vi "Create (From GObject).vi"(8 "error in (no error)":errorcluster, 10 "GObject":refnum<vi>) -> (0 "error out":errorcluster, 1 "Structure Found in":refnum<vi>, 2 "Found JKI SMs?":bool, 3 "JKI SM out":refnum<class "JKI SM.lvclass">)   [LabVIEW 2020, in "JKI State Machine API.lvlib" / "JKI SM.lvclass"]
uses:
  JKI SM.lvclass
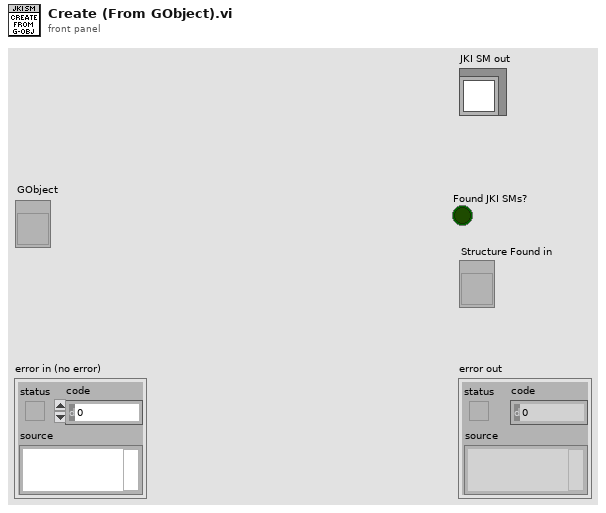
[diagram p1: front panel]
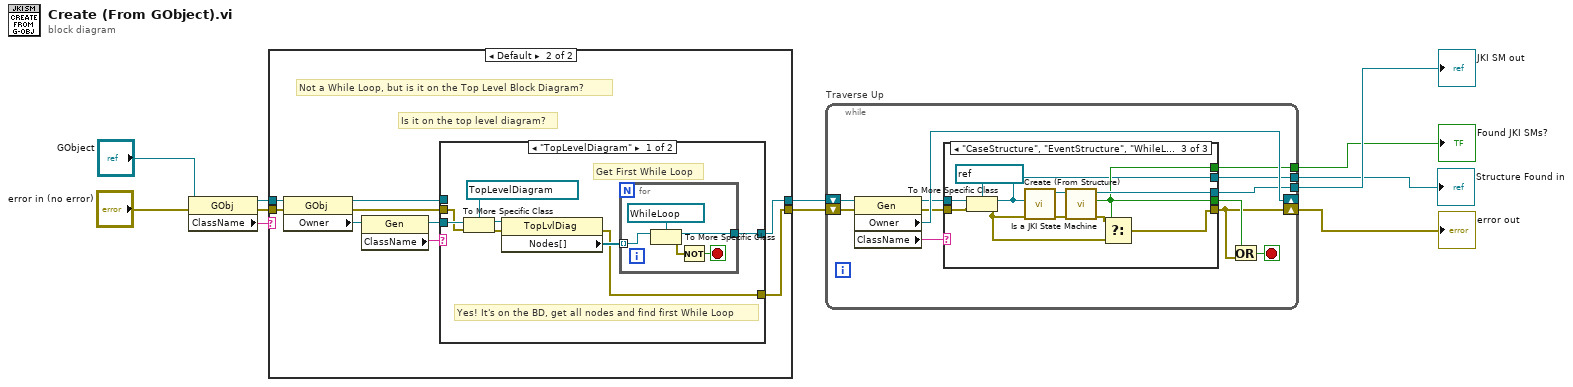
[diagram p0: block diagram]
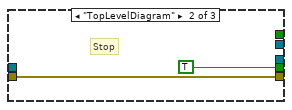
[diagram p5: hidden frame]
diagram:
  n1 = property class="GObj"(reference="GObject", error in="error in (no error)") -> (reference out=w3:refnum<vi>, error out=w2:errorcluster, "ClassName"=w1:string)
  n2 = case shown="Default" w1 {
    tunnel: [w12 w22] -> w7
    tunnel: [w13 w21] -> w6
    tunnel: w3 -> [w13 w15]
    tunnel: w2 -> [w12 w14]
    frame "WhileLoop" {
      # "It's a While Loop!\nLet's just pass it along"
    }
    frame Default {
      # "Not a While Loop, but is it on the Top Level Block Diagram?"
      # "Is it on the top level diagram?"
      n3 = property class="GObj"(reference=w15, error in=w14) -> (reference out=w20:refnum<vi>, error out=w19:errorcluster, "Owner"=w17:refnum<vi>)
      n4 = property class="Gen"(reference=w17) -> (reference out=w16:refnum<vi>, "ClassName"=w18:string)  [unwired: 1 in, 1 out]
      n5 = case shown="\"TopLevelDiagram\"" w18 {
        tunnel: w20 -> [_ w37]
        tunnel: w16 -> [w30 _]
        tunnel: [w26 w37] -> w21
        tunnel: w19 -> [w24 w36]
        tunnel: [w23 w36] -> w22
        frame "TopLevelDiagram" {
          # "Yes! It's on the BD, get all nodes and find first While Loop"
          # "Get First While Loop"
          n6 = To More Specific Class(target class=refnum<vi> refnum ("Owner"), reference=w30, error in=w24) -> (specific class reference=w28:refnum<vi>, error out=w25:errorcluster)
          n7 = property class="TopLvlDiag"(reference=w28, error in=w25) -> (error out=w23:errorcluster, "Nodes[]"=w27:refnum<vi>[])  [unwired: 1 out]
          n8 = for {
            tunnel: w27 -> [w35] mode=indexing
            tunnel: [w32] -> w26
            stop <- w31 stop-if-true
            n9 = To More Specific Class(target class=refnum<vi> refnum ("Owner"), reference=w35) -> (specific class reference=w32:refnum<vi>, error out=w33:errorcluster)  [unwired: 1 in]
            n10 = Not(x=w33) -> (.not. x?=w31:bool)
          }
        }
        frame Default {
        }
      }
    }
  }
  n11 = while "Traverse Up" {
    shift-right: [w49] -> _
    shift-left: w6 -> [w48]
    shift-right: [w40] -> w11
    shift-left: w7 -> [w44]
    tunnel: [w43] -> w10
    tunnel: [w39] -> w9
    tunnel: [w38] -> w8
    stop <- w42 stop-if-true
    n12 = property class="Gen"(reference=w48, error in=w44) -> (reference out=w46:refnum<vi>, error out=w45:errorcluster, "Owner"=w49:refnum<vi>, "ClassName"=w47:string)
    n13 = case shown="\"CaseStructure\", \"EventStructure\", \"WhileLoop\"" w47 {
      tunnel: w46 -> [_ _ w63]
      tunnel: [w50 w52 w55] -> w40
      tunnel: w45 -> [w50 w52 w61]
      tunnel: [_ _ w59] -> w43
      tunnel: [_ TRUE ("Is a JKI State Machine") w54] -> w41
      tunnel: [_ _ w54] -> w39
      tunnel: [_ _ w53] -> w38
      frame Default {
      }
      frame "TopLevelDiagram" {
        # "Stop"
      }
      frame "CaseStructure", "EventStructure", "WhileLoop" {
        n14 = To More Specific Class(target class=refnum<vi> refnum ("Structure"), reference=w63, error in=w61) -> (specific class reference=w53:refnum<vi>, error out=w56:errorcluster)
        n15 = call "Create (From Structure).vi"("error in (no error)"=w56, "Structure"=w53) -> ("error out"=w58:errorcluster, "JKI SM out"=w60:refnum<class "JKI SM.lvclass">)  [unwired: 8 in]
        n16 = call "Is a JKI State Machine.vi"("error in (no error)"=w58, "JKI SM in"=w60) -> ("error out"=w57:errorcluster, "Is a JKI State Machine"=w54:bool, "JKI SM out"=w59:refnum<class "JKI SM.lvclass">)  [unwired: 7 in]
        n17 = Select(t=w57, s=w54, f=w56) -> (s? t:f=w55:errorcluster)
      }
    }
    n18 = Or(x=w41, y=w40) -> (x .or. y?=w42:bool)
  }
  "error out" <- w11
  "JKI SM out" <- w10
  "Found JKI SMs?" <- w9
  "Structure Found in" <- w8
